vi "最小试剂余量百分比.vi"   [LabVIEW 2016, in "斯坦道CODcr.lvlib"]
uses:
  <vilib>/Analysis/BLAS.llb/izamin - Min Element Index (CDB).vi
  <vilib>/Analysis/NI_AALBLAS.lvlib
types:
  T1 = cluster{"V1":sgl, "V2":sgl, "V3":sgl, "V4":sgl, "V5":sgl, "V6":sgl, "V7":sgl, "V8":sgl, "V9":sgl, "V10":sgl, "V11":sgl, "V12":sgl, "V9-1":sgl, "V9-2":sgl}
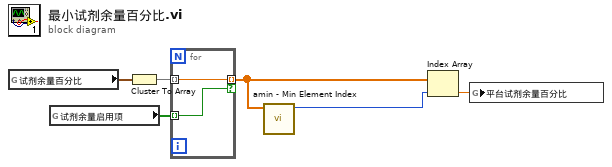
[diagram p0: block diagram]
diagram:
  n1 = global read "VAR总磷总氮全局变量.vi" "试剂余量百分比"() -> (w6:T1)
  n2 = global read "VAR总磷总氮全局变量.vi" "试剂余量启用项"() -> (w4:bool[])
  n3 = Cluster To Array(cluster=w6) -> (array=w3:sgl[])
  n4 = for {
    tunnel: w3 -> [w8] mode=indexing
    tunnel: w4 -> [w7] mode=indexing
    tunnel: [w8] -> w2 mode=indexing if=w7
  }
  n5 = call-poly <vilib>:"amin - Min Element Index.vi"("x"=w2) -> ("izamin"=w5:i32)  [unwired: 9 in, 1 out]
  n6 = Index Array(array=w2, index=w5) -> (element=w1:sgl)
  n7 = global write "VAR总磷总氮全局变量.vi" "平台试剂余量百分比"(w1) -> ()
